vi "Load_Destinations.vi"(8 "error in (no error)":errorcluster, 11 "AB_Build in":refnum<class "AB_Build.lvclass">) -> (0 "error out":errorcluster, 3 "AB_Build out":refnum<class "AB_Build.lvclass">)   [LabVIEW 2020, in "AB_Build.lvclass"]
uses:
  <vilib>/AppBuilder/AB_Classes/Build/AB_Build.lvclass
  <vilib>/AppBuilder/AB_Classes/Build/AB_Build.lvclass/AB_Build.ctl
  <vilib>/AppBuilder/AB_Classes/Destination/AB_Destination.lvclass
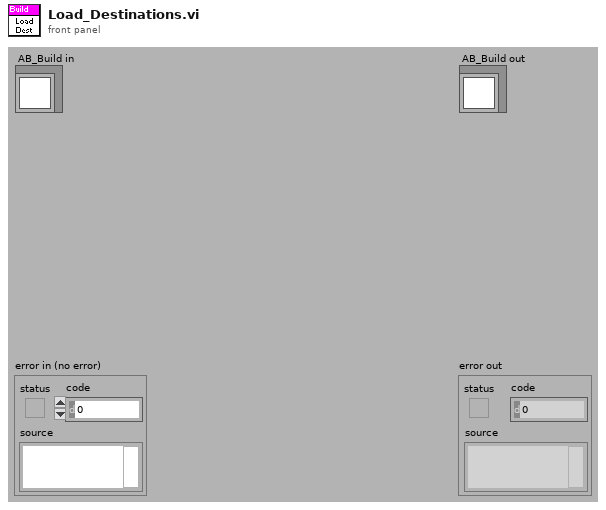
[diagram p1: front panel]
types:
  T1 = typedef "ItemRef.ctl" = u64
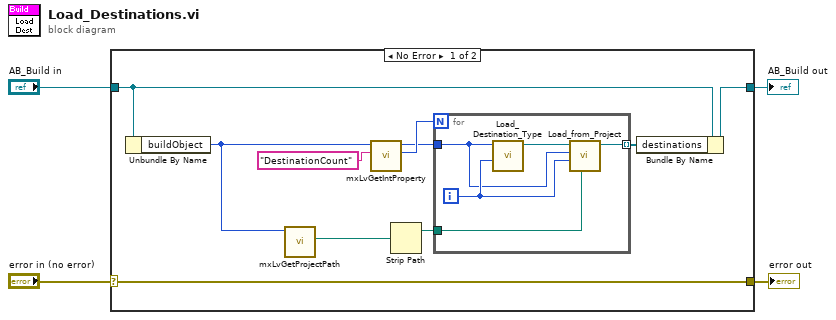
[diagram p0: block diagram]
diagram:
  n1 = case shown="No Error" "error in (no error)" {
    selector: "error in (no error)" -> [w14 w21]
    tunnel: [w14 w21] -> w3
    tunnel: [w12 w20] -> w1
    tunnel: "AB_Build in" -> [w13 w20]
    frame No Error {
      n2 = Unbundle By Name(w13) -> ("buildObject"=w6:T1)
      n3 = call <resource>:"mxLvGetProjectPath.vi"("Item"=w6) -> ("Project Path"=w5:path)  [unwired: 8 in, 2 out]
      n4 = call <resource>:"mxLvGetIntProperty.vi"("Tag"="DestinationCount", "Item"=w6) -> ("Value"=w10:i32, "Item"=w9:T1)  [unwired: 7 in, 1 out]
      n5 = Strip Path(path=w5) -> (stripped path=w7:path)  [unwired: 1 out]
      n6 = for {
        N: w10 -> [_]
        tunnel: w9 -> [w17]
        tunnel: [w16] -> w8 mode=indexing
        tunnel: w7 -> [w15]
        i -> [w18]
        n7 = call <vilib>:"Load_Destination_Type.vi"("index"=w18, "buildObject"=w17) -> ("AB_Destination out"=w19:refnum<class "AB_Destination.lvclass">)  [unwired: 8 in, 1 out]
        n8 = call-dynamic "Load_from_Project.vi"("commonPath"=w15, "index"=w18, "buildObject"=w17, "AB_Destination in"=w19) -> ("AB_Destination out"=w16:refnum<class "AB_Destination.lvclass">)  [unwired: 6 in, 1 out]
      }
      n9 = Bundle By Name(cluster=w13, "destinations"=w8) -> (w12:refnum<class "AB_Build.lvclass">)
    }
    frame Error {
    }
  }
  "error out" <- w3
  "AB_Build out" <- w1
